vi "convertToKeyValuePair_2Ddouble.vi"(8 "error in (no error)":errorcluster, 9 "presicion (0)":u8, 10 "value":dbl[][](array[numeric])=[[1.2, 0.3]], 11 "name":string) -> (0 "error out":errorcluster, 3 "string converted":string)   [LabVIEW 2018]
doc: "Convert a 2-dimension double array into a key value pair as string."
uses:
  convertToKeyValuePair_string.vi
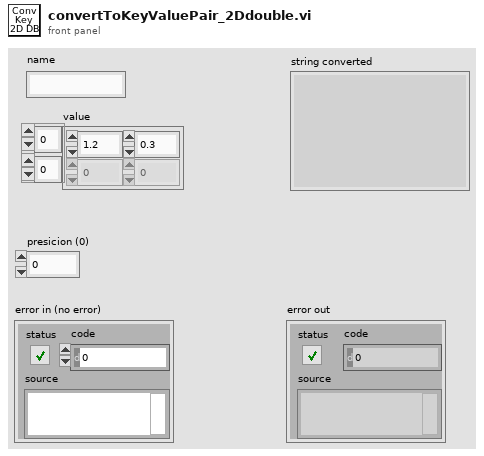
[diagram p1: front panel]
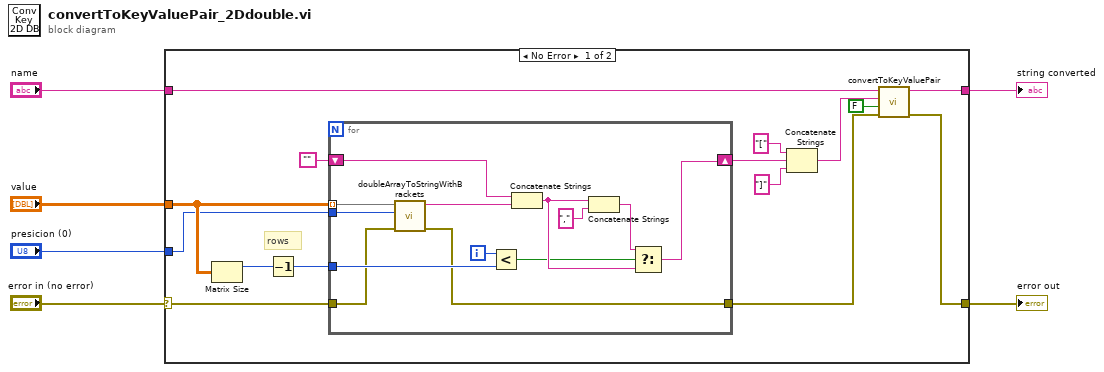
[diagram p0: block diagram]
diagram:
  n1 = case shown="No Error" "error in (no error)" {
    selector: "error in (no error)" -> [w13 w35]
    tunnel: [w11 _] -> w6
    tunnel: "name" -> [w12 _]
    tunnel: [w8 w35] -> w3
    tunnel: "value" -> [w19 _]
    tunnel: "presicion (0)" -> [w14 _]
    frame No Error {
      # "rows"
      n2 = Matrix Size(0:w19) -> (1:w18:i32)  [unwired: 1 out]
      n3 = Decrement(x=w18) -> (x-1=w17:i32)
      n4 = for {
        tunnel: w19 -> [w26] mode=indexing
        tunnel: w17 -> [w27]
        shift-right: [w29] -> w15
        shift-left: "" -> [w30]
        tunnel: w14 -> [w25]
        tunnel: w13 -> [w23]
        tunnel: [w22] -> w9
        i -> [w28]
        n5 = call "doubleArrayToStringWithBrackets.vi"("error in (no error)"=w23, "presicion (0)"=w25, "value"=w26) -> ("error out"=w22:errorcluster, "String"=w24:string)  [unwired: 7 in]
        n6 = Less?(x=w28, y=w27) -> (x < y?=w32:bool)
        n7 = Concatenate Strings(w30, w24) -> (w34:string)
        n8 = Concatenate Strings(w34, ",") -> (w33:string)
        n9 = Select(t=w33, s=w32, f=w34) -> (s? t:f=w29:string)
      }
      n10 = Concatenate Strings("[" ("string"), w15, "]" ("string")) -> (w10:string)
      n11 = call-poly "convertToKeyValuePair.vi"("error in (no error)"=w9, "double quotes (T)"=FALSE, "value"=w10, "name"=w12) -> ("error out"=w8:errorcluster, "string converted"=w11:string)  [unwired: 6 in]
    }
    frame Error {
    }
  }
  "error out" <- w3
  "string converted" <- w6
